vi "2.vi"() -> ()   [LabVIEW 2017]
panel:
  out "波形图":dbl[](graph)
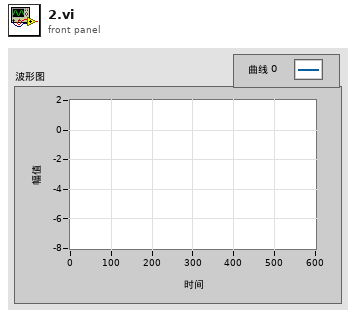
[diagram p1: front panel]
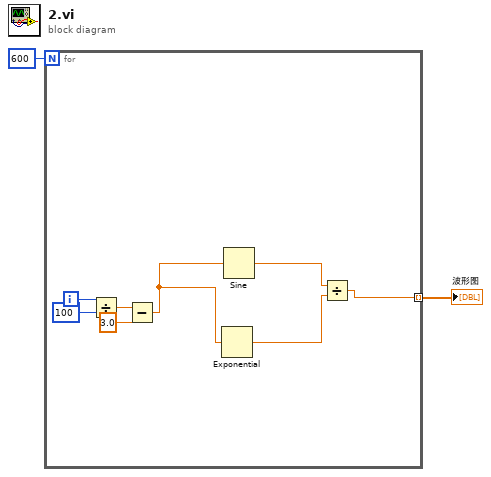
[diagram p0: block diagram]
diagram:
  n1 = for {
    N: 600 -> [_]
    tunnel: [w3] -> w1 mode=indexing
    i -> [w10]
    n2 = Divide(x=w10, y=100) -> (x/y=w8:dbl)
    n3 = Subtract(x=w8, y=3.0) -> (x-y=w6:dbl)
    n4 = Exponential(1:w6) -> (0:w4:dbl)
    n5 = Sine(x=w6) -> (sin(x)=w5:dbl)
    n6 = Divide(x=w5, y=w4) -> (x/y=w3:dbl)
  }
  "波形图" <- w1
